vi "Close.vi"(8 "error in (no error)":errorcluster caption="entrée d'erreur (pas d'erreur)", 11 "Class CSV_File (Default) en entrée":refnum<class "Class File (Default).lvclass">) -> (0 "error out":errorcluster caption="sortie d'erreur", 3 "Class CSV_File (Default) en sortie":refnum<class "Class File (Default).lvclass">)   [LabVIEW 2020, in "Library Instrument & Equipement.lvlib" / "Library File.lvlib" / "Class File (Default).lvclass"]
uses:
  Class File (Default).lvclass
  Class File (Default).lvclass/Class File (Default).ctl
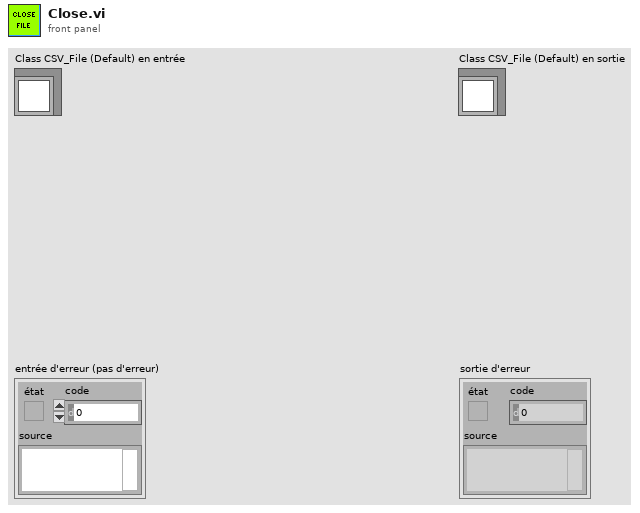
[diagram p1: front panel]
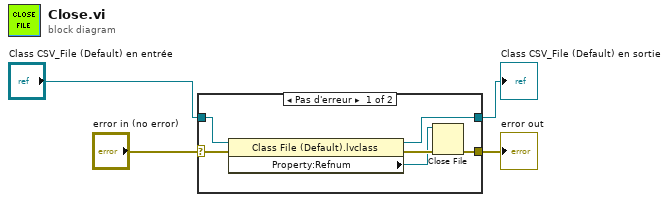
[diagram p0: block diagram]
diagram:
  n1 = case shown="Pas d'erreur" "error in (no error)" {
    selector: "error in (no error)" -> [w7 w12]
    tunnel: [w6 w12] -> w3
    tunnel: [w9 w11] -> w1
    tunnel: "Class CSV_File (Default) en entrée" -> [w10 w11]
    frame No Error {
      n2 = property class="Class File (Default).lvclass"(reference=w10, error in=w7) -> (reference out=w9:refnum<class "Class File (Default).lvclass">, error out=w8:errorcluster, "Property:Refnum"=w5:refnum<file>)
      n3 = Close File(refnum=w5, error in=w8) -> (error out=w6:errorcluster)  [unwired: 1 out]
    }
    frame Error {
    }
  }
  "error out" <- w3
  "Class CSV_File (Default) en sortie" <- w1
